vi "TriggerConfigurationGlobal.vi"(7 "Action":T8, 11 "Set Value":T1={"Arm"={"Source"=enum."Hold", "Count"=1, "Infinite?"=FALSE}, "Scan"={"Source"=enum."Hold", "Count"=0, "Infinite?"=FALSE, "Delay (sec)"=0.0, "Interval (sec)"=0.0}, "Channel"={"Source"=enum."Hold", "Count"=0, "Infinite?"=FALSE, "Auto Count?"=FALSE, "Delay (sec)"=0.0, "Interval (sec)"=0.0}} {"Arm"."Count" min=1 max=99999 step=1}) -> (3 "Value Out":T1={"Arm"={"Source"=enum."Hold", "Count"=1, "Infinite?"=FALSE}, "Scan"={"Source"=enum."Hold", "Count"=0, "Infinite?"=FALSE, "Delay (sec)"=0.0, "Interval (sec)"=0.0}, "Channel"={"Source"=enum."Hold", "Count"=0, "Infinite?"=FALSE, "Auto Count?"=FALSE, "Delay (sec)"=0.0, "Interval (sec)"=0.0}} {"Arm"."Count" min=1 max=99999 step=1})   [LabVIEW 2012]
uses:
  TriggerConfigurationGlobalAction.ctl
  TriggerConfiguration.ctl
  TriggerArmConfiguration.ctl
  driver/Public/Controls/ArmSource.ctl
  TriggerScanConfiguration.ctl
  driver/Public/Controls/ScanSource.ctl
  TriggerChannelConfiguration.ctl
  driver/Public/Controls/TriggerSource.ctl
  driver/Keithley-7001.lvlib
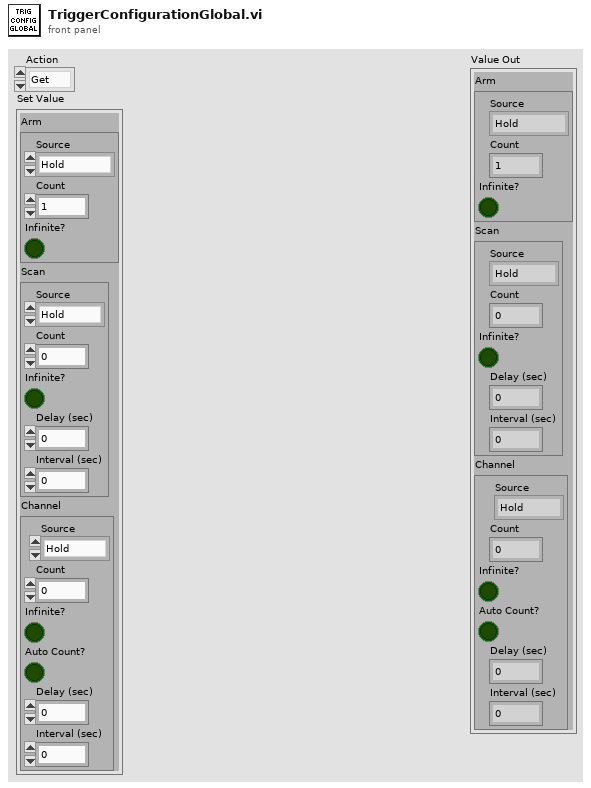
[diagram p1: front panel]
types:
  T1 = typedef "TriggerConfiguration.ctl" = cluster{"Arm":T2, "Scan":T4, "Channel":T6}
  T2 = typedef "TriggerArmConfiguration.ctl" = cluster{"Source":T3, "Count":u32, "Infinite?":bool}
  T3 = typedef "Keithley-7001.lvlib/ArmSource.ctl" = enum16{"Hold", "Immediate", "Manual", "Bus", "TLink", "External"}
  T4 = typedef "TriggerScanConfiguration.ctl" = cluster{"Source":T5, "Count":u32, "Infinite?":bool, "Delay (sec)":dbl, "Interval (sec)":dbl}
  T5 = typedef "Keithley-7001.lvlib/ScanSource.ctl" = enum16{"Hold", "Immediate", "Timer", "Manual", "Bus", "TLink", "External"}
  T6 = typedef "TriggerChannelConfiguration.ctl" = cluster{"Source":T7, "Count":u32, "Infinite?":bool, "Auto Count?":bool, "Delay (sec)":dbl, "Interval (sec)":dbl}
  T7 = typedef "Keithley-7001.lvlib/TriggerSource.ctl" = enum16{"Hold", "Immediate", "Manual", "Bus", "TLink", "External", "Timer"}
  T8 = typedef "TriggerConfigurationGlobalAction.ctl" = enum16{"Get", "Set", "Reset"}
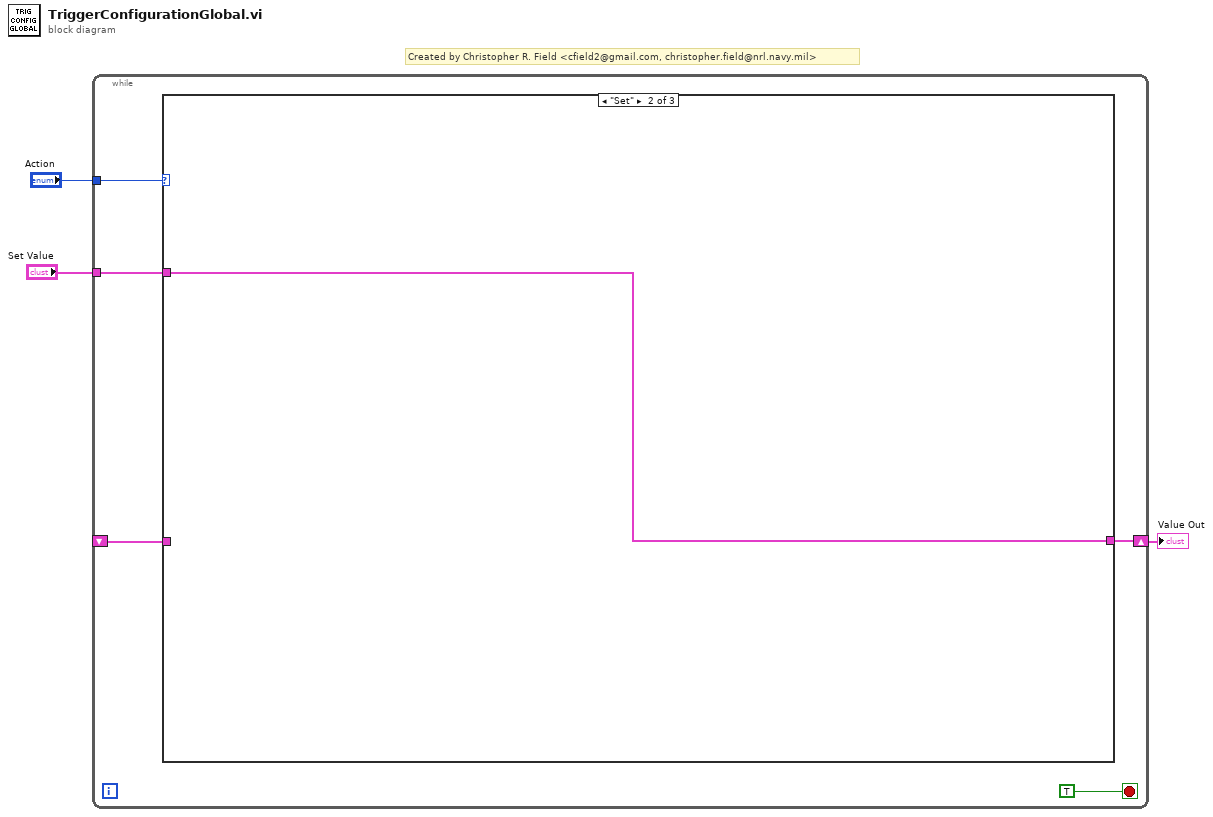
[diagram p0: block diagram]
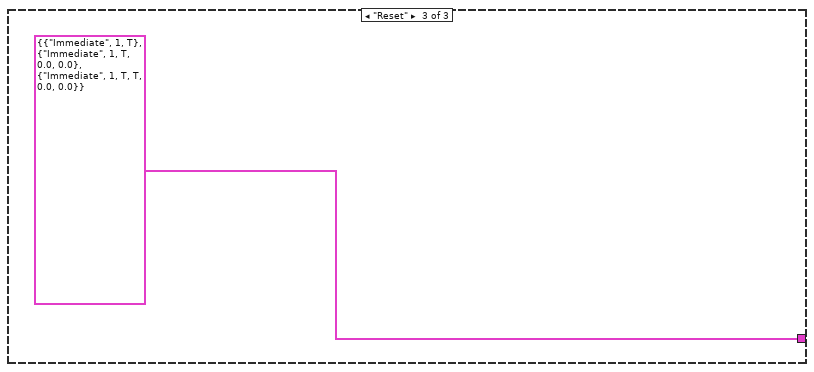
[diagram p3: hidden frame]
diagram:
  # "Created by Christopher R. Field <cfield2@gmail.com, christopher.field@nrl.navy.mil>"
  n1 = while {
    tunnel: "Action" -> [w8]
    shift-right: [w6] -> w1
    shift-left: _ -> [w5]
    tunnel: "Set Value" -> [w4]
    stop <- TRUE stop-if-true
    n2 = case shown="\"Set\"" w8 {
      tunnel: [w9 w10 T1 {"Arm"={"Source"=enum."Immediate", "Count"=1, "Infinite?"=TRUE}, "Scan"={"Source"=enum."Immediate", "Count"=1, "Infinite?"=TRUE, "Delay (sec)"=0.0, "Interval (sec)"=0.0}, "Channel"={"Source"=enum."Immediate", "Count"=1, "Infinite?"=TRUE, "Auto Count?"=TRUE, "Delay (sec)"=0.0, "Interval (sec)"=0.0}} ("Trigger Configuration")] -> w6
      tunnel: w5 -> [w9 _ _]
      tunnel: w4 -> [_ w10 _]
      frame "Get", Default {
      }
      frame "Set" {
      }
      frame "Reset" {
      }
    }
  }
  "Value Out" <- w1
